vi "UI_AutoRefresh_Do.vi"(8 "error in (no error)":errorcluster, 9 "Parameters":T1={"Write TipStrips with details (T)"=TRUE, "Write Captions with UserLabels (T)"=TRUE, "Mode (ind only)"=enum."Indicators only", "Enable nested stream (T)"=TRUE}, 10 "Databox_sealed":refnum<class "Databox_sealed.lvclass">, 11 "UIA_ChildTest in":refnum<class "UIA_ChildTest.lvclass">) -> (0 "error out":errorcluster, 3 "UIA_ChildTest out":refnum<class "UIA_ChildTest.lvclass">)   [LabVIEW 2020, in "UIA_ChildTest.lvlib" / "UIA_ChildTest.lvclass"]
uses:
  UIA_ChildTest.lvclass
  D:/Projets/STEP AT/UI Actor/UI_Actor/UI_Actor/UI_Actor.lvclass
  support/Databox.lvlibp/Databox_sealed/Databox_sealed.lvclass
  UI_Actor/UI_Actor/ctl_AR_Parameters.ctl
  UI_Actor/UI_Actor/ctl_AR_Mode.ctl
  UI_Actor/UI_Actor/UI_Actor.lvclass
panel:
  out "DIM SysLabels":string[](array[string])
  out "Latest Data":dbl[](array[numeric])
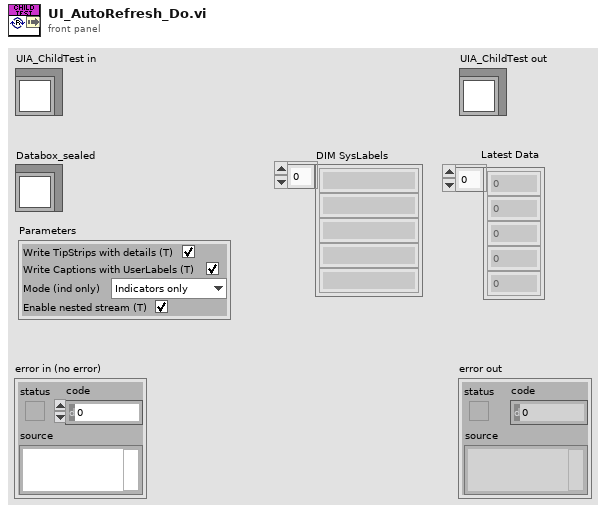
[diagram p1: front panel]
types:
  T1 = typedef "UI_Actor.lvlib/UI_Actor.lvclass/ctl_AR_Parameters.ctl" = cluster{"Write TipStrips with details (T)":bool, "Write Captions with UserLabels (T)":bool, "Mode (ind only)":T2, "Enable nested stream (T)":bool}
  T2 = typedef "UI_Actor.lvlib/UI_Actor.lvclass/ctl_AR_Mode.ctl" = enum16{"Controls only", "Indicators only", "All"}
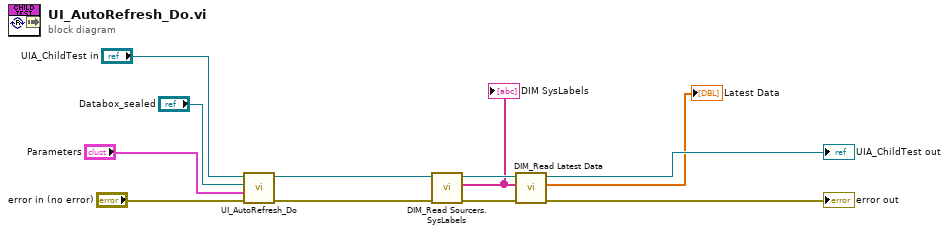
[diagram p0: block diagram]
diagram:
  n1 = call-parent "UI_AutoRefresh_Do.vi"("error in (no error)"="error in (no error)", "Parameters"="Parameters", "Databox_sealed"="Databox_sealed", "UI_Actor in"="UIA_ChildTest in") -> ("error out"=w4:errorcluster, "UI_Actor out"=w5:refnum<class "UIA_ChildTest.lvclass">)  [unwired: 6 in]
  n2 = call "DIM_Read Sourcers.SysLabels.vi"("error in (no error)"=w4, "UI_Actor in"=w5) -> ("error out"=w2:errorcluster, "DIM Sourcer.SysLabels"=w1:string[], "UI_Actor out"=w3:refnum<class "UIA_ChildTest.lvclass">)  [unwired: 7 in]
  "DIM SysLabels" <- w1
  n3 = call "DIM_Read Latest Data.vi"("error in (no error)"=w2, "Src.SysLabels"=w1, "UI_Actor in"=w3) -> ("error out"=→"error out":errorcluster, "Latest Data"=→"Latest Data":dbl[], "UI_Actor out"=→"UIA_ChildTest out":refnum<class "UIA_ChildTest.lvclass">)  [unwired: 6 in]
